vi "dfd_CIC_OutputU.vi"(10 "input valid":bool, 11 "input data":bool[](array[boolean])) -> (2 "output valid":bool, 3 "output data":fxp<+/-,32,32>)   [LabVIEW 2017]
uses:
  <vilib>/rvi/FXPMathLib/FxpMul/XNode/nifxpmath_Multiplier.xnode
  <vilib>/rvi/FXPMathLib/sim/FxpSim.dll
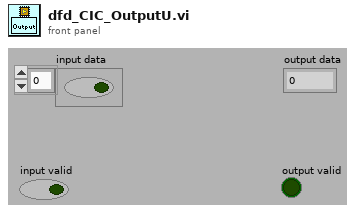
[diagram p1: front panel]
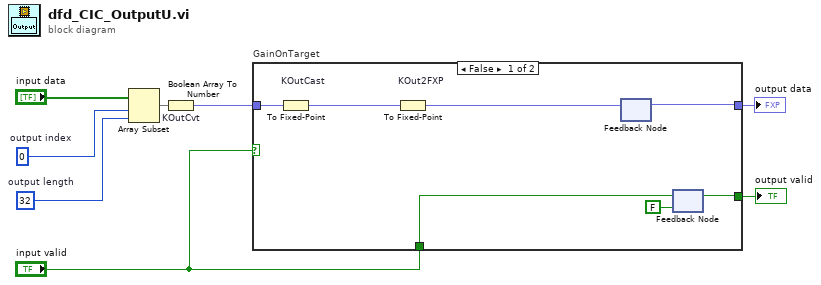
[diagram p0: block diagram]
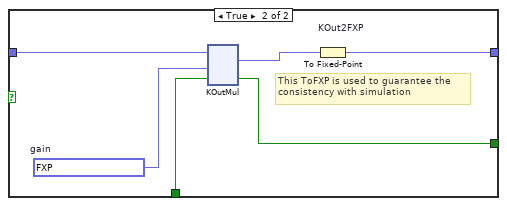
[diagram p2: hidden frame]
diagram:
  w4 = 32  # output length
  w5 = 0  # output index
  n1 = Array Subset(array="input data", index=w5, length=w4) -> (w2:bool[])
  n2 = Boolean Array To Number "KOutCvt"(Boolean array=w2) -> (number=w6:fxp<+/-,32,32>)
  n3 = case "GainOnTarget" shown="False" "input valid" {
    tunnel: "input valid" -> [w13 w21]
    tunnel: [w12 w20] -> w8
    tunnel: [w14 w18] -> w7
    tunnel: w6 -> [w11 w16]
    frame False {
      n4 = To Fixed-Point "KOutCast"(number=w11) -> (fixed-point=w9:fxp<+/-,32,32>)  [unwired: 1 in]
      n5 = To Fixed-Point "KOut2FXP"(number=w9) -> (fixed-point=w10:fxp<+/-,32,32>)  [unwired: 1 out]
      n6 = feedback-in #1(w10) -> ()
      n7 = feedback #1() -> (w14:fxp<+/-,32,32>)  [unwired: 1 out]
      n8 = feedback-in #2(w13) -> ()
      n9 = feedback #2(FALSE ("input valid")) -> (w12:bool)
    }
    frame True {
      w19 = fxp<+/-,16,1> 0.999969482421875  # gain
      # "This ToFXP is used to guarantee the \nconsistency with simulation"
      n10 = xnode "KOutMul"("x"=w16, "y"=w19, "input valid"=w21) -> ("x*y"=w17:fxp<+/-,32,32>, "output valid"=w20:bool)  [unwired: 1 in, 1 out]
      n11 = To Fixed-Point "KOut2FXP"(number=w17) -> (fixed-point=w18:fxp<+/-,32,32>)  [unwired: 1 out]
    }
  }
  "output valid" <- w8
  "output data" <- w7
